vi "RT Driver VI.vi"(7 "Operation":T1, 11 "Device Reference in":T2 format="%.0x") -> (0 "Error Code":i32)   [LabVIEW 2019, in "MD4Logger Engine.lvlib"]
uses:
  MD4Logger Engine.lvlib
  <vilib>/NI VeriStand/Custom Device API/Custom Device Item Ref.ctl
  <vilib>/NI VeriStand/Custom Device API/Hardware Interface Driver VI Operation.ctl
  Shared/Compiled.Settings.ctl
  RTStateVariables.ctl
  <vilib>/NI/NIVS Inline Async API/_VS Inline Async API/VS Inline Async API/VS Inline Async API.lvclass
  <vilib>/NI VeriStand/Custom Device API/Custom Device Channel Type.ctl
  <vilib>/NI/NIVS Inline Async API/_VS Inline Async API/VS Inline Async API/VS Inline Async API.lvclass/VS Inline Async API.ctl
  <vilib>/NI/NIVS Inline Async API/_Data Access Engine/Data Access Engine/Data Access Engine.lvclass/Data Access Engine.ctl
  <vilib>/NI/NIVS Inline Async API/_Data Access Engine/Access Type Classes/Write/Write.lvclass/Write.ctl
  <vilib>/NI/NIVS Inline Async API/_Data Access Engine/Access Type Classes/ReadWrite/ReadWrite.lvclass/ReadWrite.ctl
  <vilib>/NI/NIVS Inline Async API/_Data Access Engine/Access Type Classes/Read/Read.lvclass/Read.ctl
  <vilib>/NI/NIVS Inline Async API/_Data Access Engine/Data Access Engine/Methods/Data.Engine.Read Data from HW.vi
  <vilib>/NI/NIVS Inline Async API/_VS Inline Async API/Error Handling Process/SubVIs/Error.GetError.vi
  <vilib>/NI/NIVS Inline Async API/_Data Access Engine/Data Access Engine/Methods/Data.Engine.Write Data to HW.vi
  <vilib>/NI/NIVS Inline Async API/_Data Access Engine/Access Type Classes/ReadWrite/ReadWrite.EngineData.vi
  <vilib>/NI/NIVS Inline Async API/_Data Access Engine/Access Type Classes/Write/Write.EngineData.vi
  <vilib>/NI/NIVS Inline Async API/_Data Access Engine/Access Type Classes/Read/Read.EngineData.vi
  <vilib>/NI VeriStand/Custom Device API/NI VeriStand - Get Channel Value by Data Reference.vi
  <vilib>/NI VeriStand/Custom Device API/NI VeriStand - Set Channel Value by Data Reference.vi
  <vilib>/NI VeriStand/Custom Device API/NI VeriStand - Get Channel Values by Block Data Reference.vi
  Shared/Constants.vi
  <vilib>/NI VeriStand/Custom Device Tools/Custom Device Utility Library/NI VeriStand - Search for Item by GUID.vi
  <vilib>/NI VeriStand/Custom Device API/Get Item Property (Path).vi
  <vilib>/NI VeriStand/Custom Device API/Get Item Property (String).vi
  <vilib>/NI VeriStand/Custom Device API/Global Data Refs.vi
  <vilib>/NI VeriStand/Custom Device API/Custom Device API.lvlib
  <vilib>/NI VeriStand/Custom Device Tools/Custom Device Utility Library/Custom Device Utility Library.lvlib
  Shared/MD4Logger Shared.lvlib
  <vilib>/NI VeriStand/Custom Device API/Set Item Property (Variant).vi
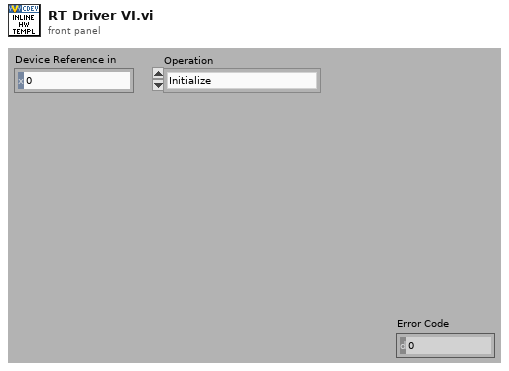
[diagram p1: front panel]
types:
  T1 = typedef "Custom Device API.lvlib/Hardware Interface Driver VI Operation.ctl" = enum16{"Initialize", "Start", "Read Data from HW", "Write Data to HW", "Close"}
  T2 = typedef "Custom Device API.lvlib/Custom Device Item Ref.ctl" = u64
  T3 = typedef "MD4Logger Engine.lvlib/RTStateVariables.ctl" = cluster{"Async":refnum<class "VS Inline Async API.lvclass">, "Settings":T4}
  T4 = typedef "MD4Logger Shared.lvlib/Compiled.Settings.ctl" = cluster{"Name":string, "Folder Path":path, "Channnel Names":cluster{"Name":string, "Unit":string}[], "File Name":string}
  T5 = typedef "Custom Device API.lvlib/Custom Device Channel Type.ctl" = enum16{"Input", "Output"}
  T6 = typedef "Custom Device API.lvlib/Custom Device Channel.ctl" = cluster{"Type":T5, "Units":string, "Default Value":dbl, "Faultable":bool, "Scalable":bool}
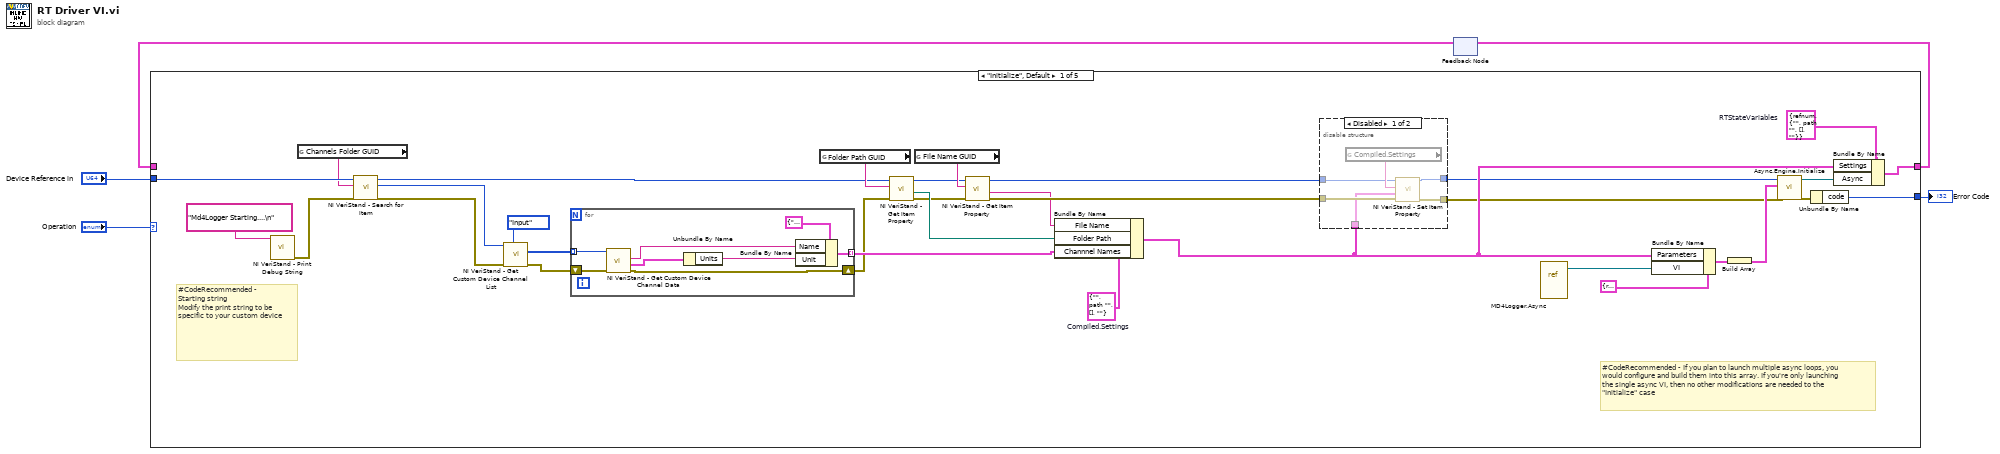
[diagram p0: block diagram]
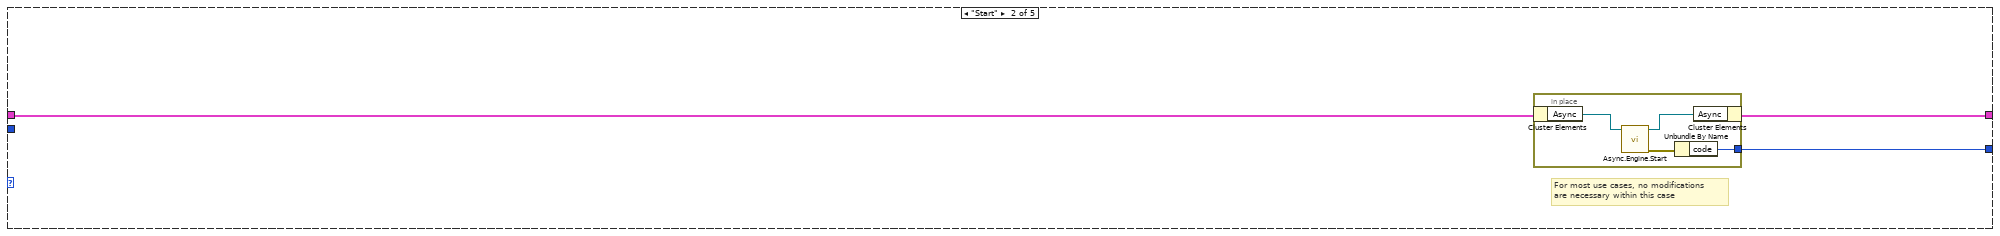
[diagram p3: hidden frame]
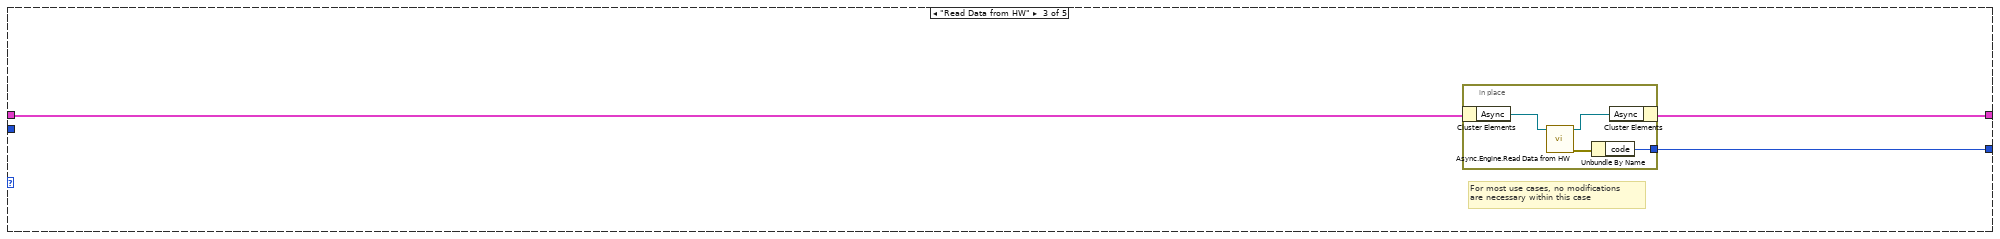
[diagram p4: hidden frame]
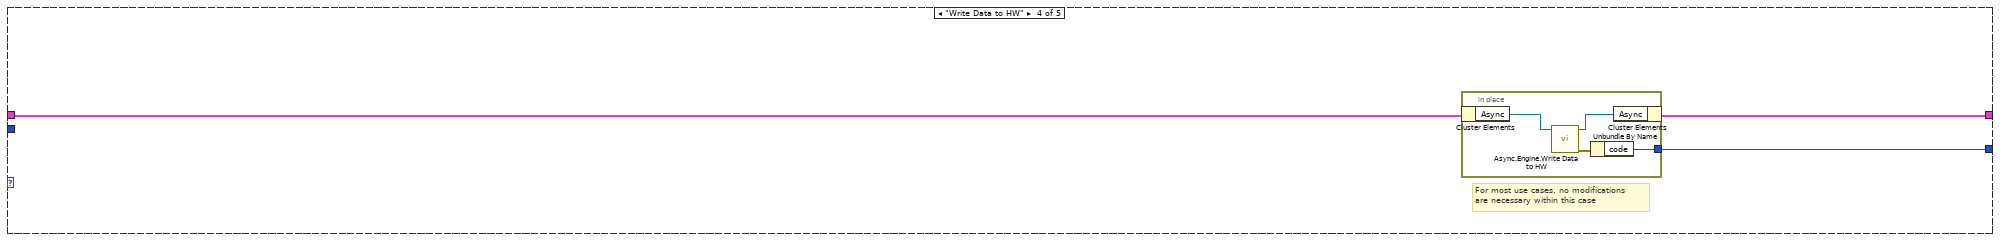
[diagram p5: hidden frame]
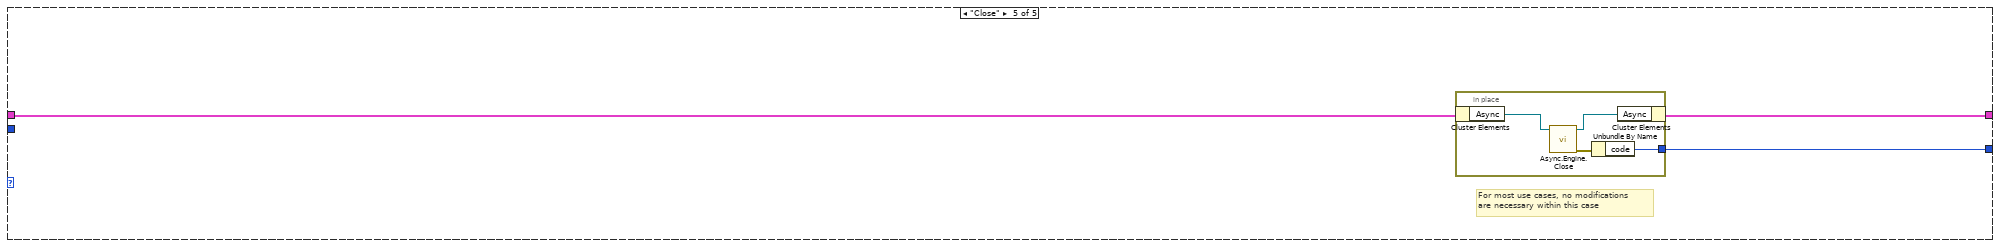
[diagram p6: hidden frame]
diagram:
  n1 = feedback #1() -> (w3:T3)  [unwired: 1 out]
  n2 = case shown="\"Initialize\", Default" "Operation" {
    tunnel: [w36 w57 w62 w69 w77] -> w4
    tunnel: w3 -> [_ w55 w64 w70 w78]
    tunnel: "Device Reference in" -> [w25 _ _ _ _]
    tunnel: [w38 w56 w63 w71 w76] -> w1
    frame "Initialize", Default {
      w32 = T3 {"Async"=refnum, "Settings"={"Name"="", "Folder Path"=path "", "Channnel Names"=[], "File Name"=""}}  # RTStateVariables
      w27 = T4 {"Name"="", "Folder Path"=path "", "Channnel Names"=[], "File Name"=""}  # Compiled.Settings
      # "#CodeRecommended - Starting string\nModify the print string to be specific to your custom device"
      # "#CodeRecommended - If you plan to launch multiple async loops, you would configure and build them into this array. If you're only launching the single async VI, then no other modifications are needed to the \"Initialize\" case"
      n3 = call <vilib>:"NI VeriStand - Print Debug String.vi"("Message"="Md4Logger Starting....\n") -> ("error out"=w14:errorcluster)  [unwired: 10 in]
      n4 = global read "Constants.vi" "Channels Folder GUID"() -> (w6:string)
      n5 = call-poly <vilib>:"NI VeriStand - Search for Item.vi"("error in"=w14, "Item GUID"=w6, "Section Ref in"=w25) -> ("error out"=w13:errorcluster, "Item Ref"=w24:T2, "Section Ref out"=w21:T2)  [unwired: 5 in, 1 out]
      n6 = call <vilib>:"NI VeriStand - Get Custom Device Channel List.vi"("Channel Type"=Custom_Device_Channel_Type."Input", "error in (no error)"=w13, "Device Ref in"=w24) -> ("error out"=w19:errorcluster, "Specified Channel Ref List"=w22:T2[])  [unwired: 6 in, 1 out]
      n7 = for {
        tunnel: w22 -> [w54] mode=indexing
        tunnel: [w51] -> w20 mode=indexing
        shift-right: [w49] -> w18
        shift-left: w19 -> [w50]
        n8 = call <vilib>:"NI VeriStand - Get Custom Device Channel Data.vi"("error in (no error)"=w50, "Channel Ref in"=w54) -> ("error out"=w49:errorcluster, "Channel"=w48:T6, "Channel Name"=w52:string)  [unwired: 4 in, 3 out]
        n9 = Unbundle By Name(w48) -> ("Units"=w47:string)
        n10 = Bundle By Name(cluster=cluster{"Name":string, "Unit":string} {"Name"="", "Unit"=""} ("Channel"), "Name"=w52, "Unit"=w47) -> (w51:cluster{"Name":string, "Unit":string})
      }
      n11 = global read "Constants.vi" "Folder Path GUID"() -> (w28:string)
      n12 = call-poly <vilib>:"NI VeriStand - Get Item Property.vi"("error in (no error)"=w18, "Property Name"=w28, "Item Ref in"=w21) -> ("error out"=w12:errorcluster, "Value"=w26:path, "Item Ref out"=w8:T2)  [unwired: 5 in, 1 out]
      n13 = global read "Constants.vi" "File Name GUID"() -> (w10:string)
      n14 = call-poly <vilib>:"NI VeriStand - Get Item Property.vi"("error in (no error)"=w12, "Property Name"=w10, "Item Ref in"=w8) -> ("error out"=w11:errorcluster, "Value"=w9:string, "Item Ref out"=w7:T2)  [unwired: 5 in, 1 out]
      n15 = Bundle By Name(cluster=w27, "File Name"=w9, "Folder Path"=w26, "Channnel Names"=w20) -> (w17:T4)
      n16 = disable-structure shown="Disabled" {
        disable-tunnel: w11 -> [w44 w45]
        disable-tunnel: w17 -> [w42 _]
        disable-tunnel: [w41 w45] -> w16
        disable-tunnel: [w40 w46] -> w15
        disable-tunnel: w7 -> [w39 w46]
        frame Disabled {
          n17 = global read "Constants.vi" "Compiled.Settings"() -> (w43:string)
          n18 = call-poly <vilib>:"NI VeriStand - Set Item Property.vi"("error in (no error)"=w44, "Value"=w42, "Property Name"=w43, "Item Ref in"=w39) -> ("error out"=w41:errorcluster, "Item Ref out"=w40:T2)  [unwired: 5 in, 1 out]
        }
        frame Enabled {
        }
      }
      n19 = vi-ref "MD4Logger.Async.vi"() -> (w29:refnum<vi>)
      n20 = Bundle By Name(cluster=cluster{"VI":refnum<vi>, "Parameters":variant} {"VI"=refnum, "Parameters"=variant} ("Process"), "Parameters"=w17, "VI"=w29) -> (w34:cluster{"VI":refnum<vi>, "Parameters":variant})
      n21 = Build Array(w34) -> (w31:cluster{"VI":refnum<vi>, "Parameters":variant}[])
      n22 = call <vilib>:"Async.Engine.Initialize.vi"("error in (no error)"=w16, "Processes"=w31, "Custom Device Ref"=w15) -> ("error out"=w33:errorcluster, "Async"=w37:refnum<class "VS Inline Async API.lvclass">)  [unwired: 7 in]
      n23 = Unbundle By Name(w33) -> ("code"=w38:i32)
      n24 = Bundle By Name(cluster=w32, "Settings"=w17, "Async"=w37) -> (w36:T3)
    }
    frame "Start" {
      # "For most use cases, no modifications \nare necessary within this case"
      n25 = in-place {
        in-place-border: [w58] -> w56
        n26 = in-place-cluster #2(w55) -> ("Async"=w61:refnum<class "VS Inline Async API.lvclass">)
        n27 = call <vilib>:"Async.Engine.Start.vi"("VS Inline Async API in"=w61) -> ("error out"=w59:errorcluster, "VS Inline Async API out"=w60:refnum<class "VS Inline Async API.lvclass">)  [unwired: 9 in]
        n28 = Unbundle By Name(w59) -> ("code"=w58:i32)
        n29 = in-place-cluster #2("Async"=w60) -> (w57:T3)
      }
    }
    frame "Read Data from HW" {
      # "For most use cases, no modifications \nare necessary within this case"
      n30 = in-place {
        in-place-border: [w66] -> w63
        n31 = in-place-cluster #3(w64) -> ("Async"=w68:refnum<class "VS Inline Async API.lvclass">)
        n32 = call <vilib>:"Async.Engine.Read Data from HW.vi"("Async in"=w68) -> ("error out"=w65:errorcluster, "Async out"=w67:refnum<class "VS Inline Async API.lvclass">)  [unwired: 9 in]
        n33 = Unbundle By Name(w65) -> ("code"=w66:i32)
        n34 = in-place-cluster #3("Async"=w67) -> (w62:T3)
      }
    }
    frame "Write Data to HW" {
      # "For most use cases, no modifications \nare necessary within this case"
      n35 = in-place {
        in-place-border: [w75] -> w71
        n36 = in-place-cluster #4(w70) -> ("Async"=w73:refnum<class "VS Inline Async API.lvclass">)
        n37 = call <vilib>:"Async.Engine.Write Data to HW.vi"("VS Inline Async API in"=w73) -> ("error out"=w74:errorcluster, "VS Inline Async API out"=w72:refnum<class "VS Inline Async API.lvclass">)  [unwired: 9 in]
        n38 = Unbundle By Name(w74) -> ("code"=w75:i32)
        n39 = in-place-cluster #4("Async"=w72) -> (w69:T3)
      }
    }
    frame "Close" {
      # "For most use cases, no modifications \nare necessary within this case"
      n40 = in-place {
        in-place-border: [w80] -> w76
        n41 = in-place-cluster #5(w78) -> ("Async"=w82:refnum<class "VS Inline Async API.lvclass">)
        n42 = call <vilib>:"Async.Engine.Close.vi"("Async in"=w82) -> ("error out"=w79:errorcluster, "Async out"=w81:refnum<class "VS Inline Async API.lvclass">)  [unwired: 9 in]
        n43 = Unbundle By Name(w79) -> ("code"=w80:i32)
        n44 = in-place-cluster #5("Async"=w81) -> (w77:T3)
      }
    }
  }
  "Error Code" <- w1
  n45 = feedback-in #1(w4) -> ()
